vi "Initialize Global Stop.vi"(8 "error in":errorcluster, 11 "Async in":refnum<class "VS Inline Async API (Express).lvclass">) -> (0 "error out":errorcluster {"code" min=0 max=0}, 3 "Async out":refnum<class "VS Inline Async API (Express).lvclass">)   [LabVIEW 2026, in "VS Inline Async API (Express).lvlib" / "VS Inline Async API (Express).lvclass"]
uses:
  VS Inline Async API (Express).lvclass
  VS Inline Async API (Express).lvclass/VS Inline Async API (Express).ctl
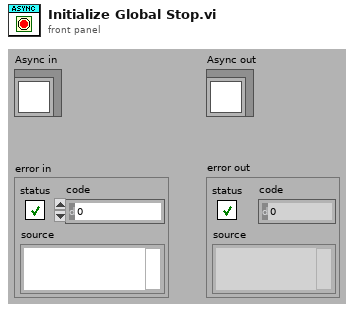
[diagram p1: front panel]
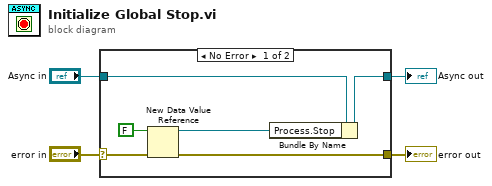
[diagram p0: block diagram]
diagram:
  n1 = case shown="No Error" "error in" {
    selector: "error in" -> [w7 w12]
    tunnel: [w6 w12] -> w4
    tunnel: "Async in" -> [w9 w11]
    tunnel: [w8 w11] -> w1
    frame No Error {
      n2 = New Data Value Reference(data value=FALSE, error in=w7) -> (data value reference=w5:refnum<data-value>, error out=w6:errorcluster)
      n3 = Bundle By Name(cluster=w9, "Process.Stop"=w5) -> (w8:refnum<class "VS Inline Async API (Express).lvclass">)
    }
    frame Error {
    }
  }
  "error out" <- w4
  "Async out" <- w1
